vi "Handle.vi"(8 "error in (no error)":errorcluster, 11 "GSserver in":refnum<class "GSserver.lvclass">) -> (0 "error out":errorcluster, 3 "GSserver out":refnum<class "GSserver.lvclass">)   [LabVIEW 2018, in "GSserver.lvclass"]
uses:
  GSserver.lvclass
  C:/Users/devstaff/sparc4/s4gui/Versao ZeroMQ REQ-REP/SPARC4_GUI -v1.0.8 - reconhecimento do ACK do ACS/Server/Server.lvclass
  GSserver.lvclass/GSserver.ctl
  Device/Device.lvclass/Device.ctl
  Server/Server.lvclass/Server.ctl
  GSstatus/GSstatus.lvclass
  C:/Users/devstaff/sparc4/s4gui/Versao ZeroMQ REQ-REP/SPARC4_GUI -v1.0.8 - reconhecimento do ACK do ACS/Device/Device.lvclass
  Server/Server.lvclass
  Comm/Stream/Stream.lvclass
  GSdevice/GSdevice.lvclass
  Device/Device.lvclass
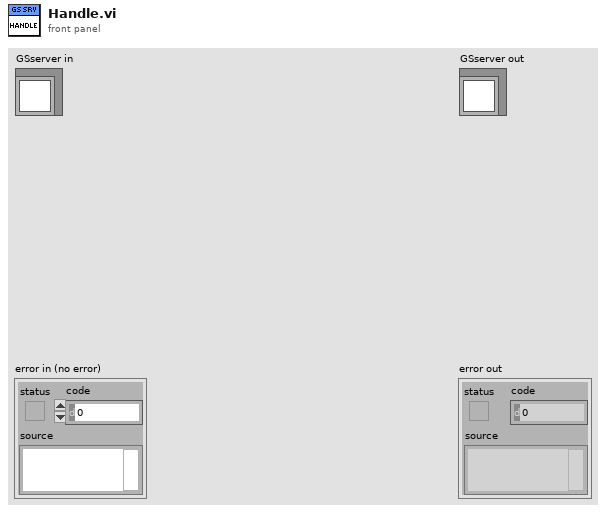
[diagram p1: front panel]
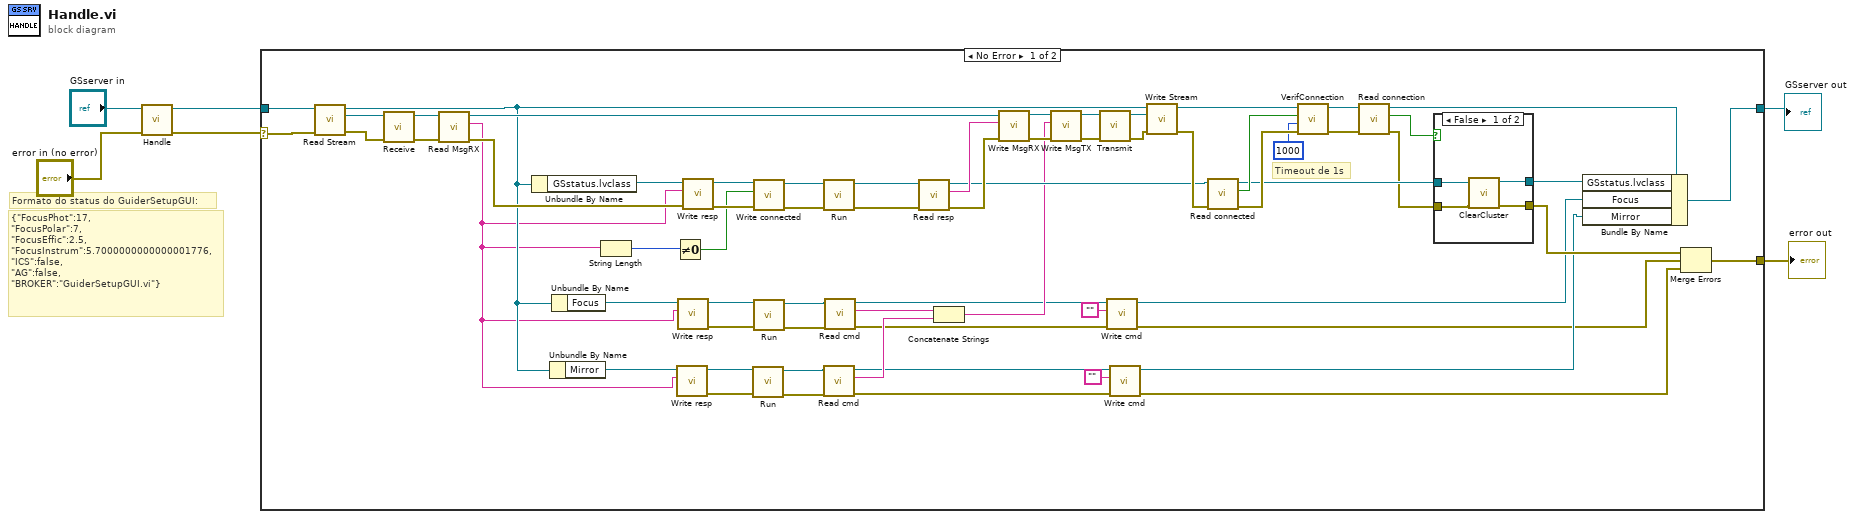
[diagram p0: block diagram]
diagram:
  # "Formato do status do GuiderSetupGUI:"
  # "{\"FocusPhot\":17,\n\"FocusPolar\":7,\n\"FocusEffic\":2.5,\n\"FocusInstrum\":5.7000000000000001776,\n\"ICS\":false,\n\"AG\":false,\n\"BROKER\":\"GuiderSetupGUI.vi\"}"
  n1 = call-parent "Handle.vi"("error in (no error)"="error in (no error)", "Server in"="GSserver in") -> ("error out"=w3:errorcluster, "Server out"=w4:refnum<class "GSserver.lvclass">)  [unwired: 8 in]
  n2 = case shown="No Error" w3 {
    selector: w3 -> [w70 w80]
    tunnel: [w17 w80] -> w2
    tunnel: [w69 w79] -> w1
    tunnel: w4 -> [w65 w79]
    frame No Error {
      # "Timeout de 1s"
      n3 = call-dynamic "Read Stream.vi"("error in (no error)"=w70, "Server in"=w65) -> ("error out"=w71:errorcluster, "Stream.lvclass"=w72:refnum<class "Stream.lvclass">, "Server out"=w23:refnum<class "GSserver.lvclass">)  [unwired: 7 in]
      n4 = call-dynamic "Receive.vi"("error in (no error)"=w71, "Stream in"=w72) -> ("error out"=w68:errorcluster, "Stream out"=w67:refnum<class "Stream.lvclass">)  [unwired: 8 in]
      n5 = call-dynamic "Read MsgRX.vi"("error in (no error)"=w68, "Comm in"=w67) -> ("error out"=w66:errorcluster, "MsgRX"=w22:string, "Comm out"=w48:refnum<class "Stream.lvclass">)  [unwired: 7 in]
      n6 = Unbundle By Name(w23) -> ("GSstatus.lvclass"=w58:refnum<class "GSstatus.lvclass">)
      n7 = Unbundle By Name(w23) -> ("Mirror"=w28:refnum<class "GSdevice.lvclass">)
      n8 = Unbundle By Name(w23) -> ("Focus"=w33:refnum<class "GSdevice.lvclass">)
      n9 = String Length(string=w22) -> (length=w64:i32)
      n10 = Not Equal To 0?(x=w64) -> (x != 0?=w53:bool)
      n11 = call-dynamic "Write resp.vi"("resp"=w22, "Device in"=w28) -> ("error out"=w26:errorcluster, "Device out"=w27:refnum<class "GSdevice.lvclass">)  [unwired: 8 in]
      n12 = call-dynamic "Write resp.vi"("resp"=w22, "Device in"=w33) -> ("error out"=w31:errorcluster, "Device out"=w32:refnum<class "GSdevice.lvclass">)  [unwired: 8 in]
      n13 = call-dynamic "Write resp.vi"("error in (no error)"=w66, "resp"=w22, "Device in"=w58) -> ("error out"=w55:errorcluster, "Device out"=w57:refnum<class "GSstatus.lvclass">)  [unwired: 7 in]
      n14 = call-dynamic "Run.vi"("error in (no error)"=w26, "GSdevice in"=w27) -> ("error out"=w24:errorcluster, "GSdevice out"=w25:refnum<class "GSdevice.lvclass">)  [unwired: 8 in]
      n15 = call "Write connected.vi"("error in (no error)"=w55, "connected"=w53, "Device in"=w57) -> ("error out"=w54:errorcluster, "Device out"=w56:refnum<class "GSstatus.lvclass">)  [unwired: 7 in]
      n16 = call-dynamic "Run.vi"("error in (no error)"=w31, "GSdevice in"=w32) -> ("error out"=w29:errorcluster, "GSdevice out"=w30:refnum<class "GSdevice.lvclass">)  [unwired: 8 in]
      n17 = call-dynamic "Run.vi"("error in (no error)"=w54, "GSstatus in"=w56) -> ("error out"=w52:errorcluster, "GSstatus out"=w51:refnum<class "GSstatus.lvclass">)  [unwired: 8 in]
      n18 = call-dynamic "Read cmd.vi"("error in (no error)"=w24, "Device in"=w25) -> ("error out"=w13:errorcluster, "cmd"=w20:string, "Device out"=w14:refnum<class "GSdevice.lvclass">)  [unwired: 7 in]
      n19 = call-dynamic "Read cmd.vi"("error in (no error)"=w29, "Device in"=w30) -> ("error out"=w15:errorcluster, "cmd"=w21:string, "Device out"=w16:refnum<class "GSdevice.lvclass">)  [unwired: 7 in]
      n20 = call-dynamic "Read resp.vi"("error in (no error)"=w52, "Device in"=w51) -> ("error out"=w50:errorcluster, "resp"=w49:string, "Device out"=w47:refnum<class "GSstatus.lvclass">)  [unwired: 7 in]
      n21 = Concatenate Strings(w21, w20) -> (w19:string)
      n22 = call-dynamic "Write MsgRX.vi"("error in (no error)"=w50, "MsgRX"=w49, "Comm in"=w48) -> ("error out"=w36:errorcluster, "Comm out"=w39:refnum<class "Stream.lvclass">)  [unwired: 7 in]
      n23 = call-dynamic "Write MsgTX.vi"("error in (no error)"=w36, "MsgTX"=w19, "Comm in"=w39) -> ("error out"=w35:errorcluster, "Comm out"=w38:refnum<class "Stream.lvclass">)  [unwired: 7 in]
      n24 = call-dynamic "Transmit.vi"("error in (no error)"=w35, "Stream in"=w38) -> ("error out"=w34:errorcluster, "Stream out"=w37:refnum<class "Stream.lvclass">)  [unwired: 8 in]
      n25 = call-dynamic "Write cmd.vi"("error in (no error)"=w15, "cmd"="", "Device in"=w16) -> ("error out"=w8:errorcluster, "Device out"=w10:refnum<class "GSdevice.lvclass">)  [unwired: 7 in]
      n26 = call-dynamic "Write cmd.vi"("error in (no error)"=w13, "cmd"="", "Device in"=w14) -> ("error out"=w7:errorcluster, "Device out"=w9:refnum<class "GSdevice.lvclass">)  [unwired: 7 in]
      n27 = call-dynamic "Write Stream.vi"("error in (no error)"=w34, "Stream.lvclass"=w37, "Server in"=w23) -> ("error out"=w63:errorcluster, "Server out"=w62:refnum<class "GSserver.lvclass">)  [unwired: 7 in]
      n28 = call "Read connected.vi"("error in (no error)"=w63, "Device in"=w47) -> ("error out"=w60:errorcluster, "connected"=w61:bool, "Device out"=w42:refnum<class "GSstatus.lvclass">)  [unwired: 7 in]
      n29 = call-dynamic "VerifConnection.vi"("error in (no error)"=w60, "timeout in ms (1000)"=u32 1000 ("period (ms)"), "device connected in"=w61, "Server in"=w62) -> ("error out"=w44:errorcluster, "Server out"=w45:refnum<class "GSserver.lvclass">)  [unwired: 6 in]
      n30 = call "Read connection.vi"("error in (no error)"=w44, "Server in"=w45) -> ("error out"=w40:errorcluster, "connection"=w46:bool, "Server out"=w43:refnum<class "GSserver.lvclass">)  [unwired: 7 in]
      n31 = case shown="False" w46 {
        tunnel: [w75 w78] -> w41
        tunnel: w42 -> [w76 w78]
        tunnel: w40 -> [w74 w77]
        tunnel: [w73 w77] -> w18
        frame False {
          n32 = call-dynamic "ClearCluster.vi"("error in (no error)"=w74, "GSstatus in"=w76) -> ("error out"=w73:errorcluster, "GSstatus out"=w75:refnum<class "GSstatus.lvclass">)  [unwired: 8 in]
        }
        frame True {
        }
      }
      n33 = Bundle By Name(cluster=w43, "GSstatus.lvclass"=w41, "Focus"=w10, "Mirror"=w9) -> (w69:refnum<class "GSserver.lvclass">)
      n34 = Merge Errors(w18, w8, w7) -> (w17:errorcluster)
    }
    frame Error {
    }
  }
  "error out" <- w2
  "GSserver out" <- w1
